vi "test_RK110512Fiber_Spiral.vi"() -> ()   [LabVIEW 2010, in "FPGAWrapperRK110512Fiber_Spiral.lvclass"]
uses:
  FPGAWrapperRK110512Fiber_Spiral.lvclass
  common/arrays/pixel_raw_data_array.ctl
panel:
  out "DAQ loop counter":i32
  out "channel data block":dbl[][](graph)
  out "timed out?":bool
  in  "timeout (ms)":i32
  in  "block size":i32
  in  "number of channels":i32
  out "Pixel dwell time":dbl
  in  "Run":bool
  in  "Cycles per pixel":i32
  in  "Create":bool
  out "FPGAWrapper out":refnum<class "FPGAWrapperRK110512Fiber_Spiral.lvclass">
  in  "Stop":bool
  # "Test VI for FPGAWrapperRK110512Fiber_Spiral"
  # "µs"
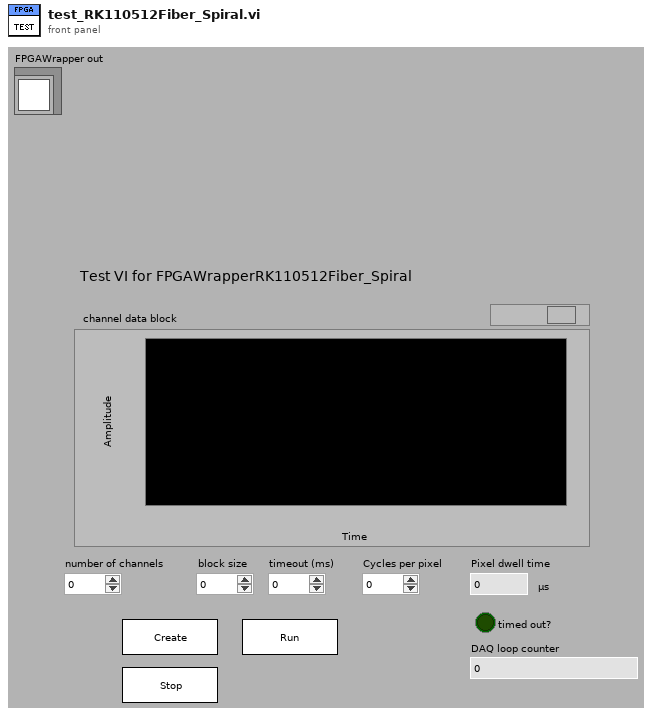
[diagram p1: front panel]
types:
  T1 = typedef "plugin_specification.ctl" = cluster{"class path":string, "configuration":string, "label":string, "settings name":string}
  T2 = typedef "XComponentSpecification.xctl/data.ctl" = cluster{"class path":string, "configuration":string, "label":string, "settings name":string}
  T3 = typedef "pixel_raw_data_array.ctl" = dbl[][]
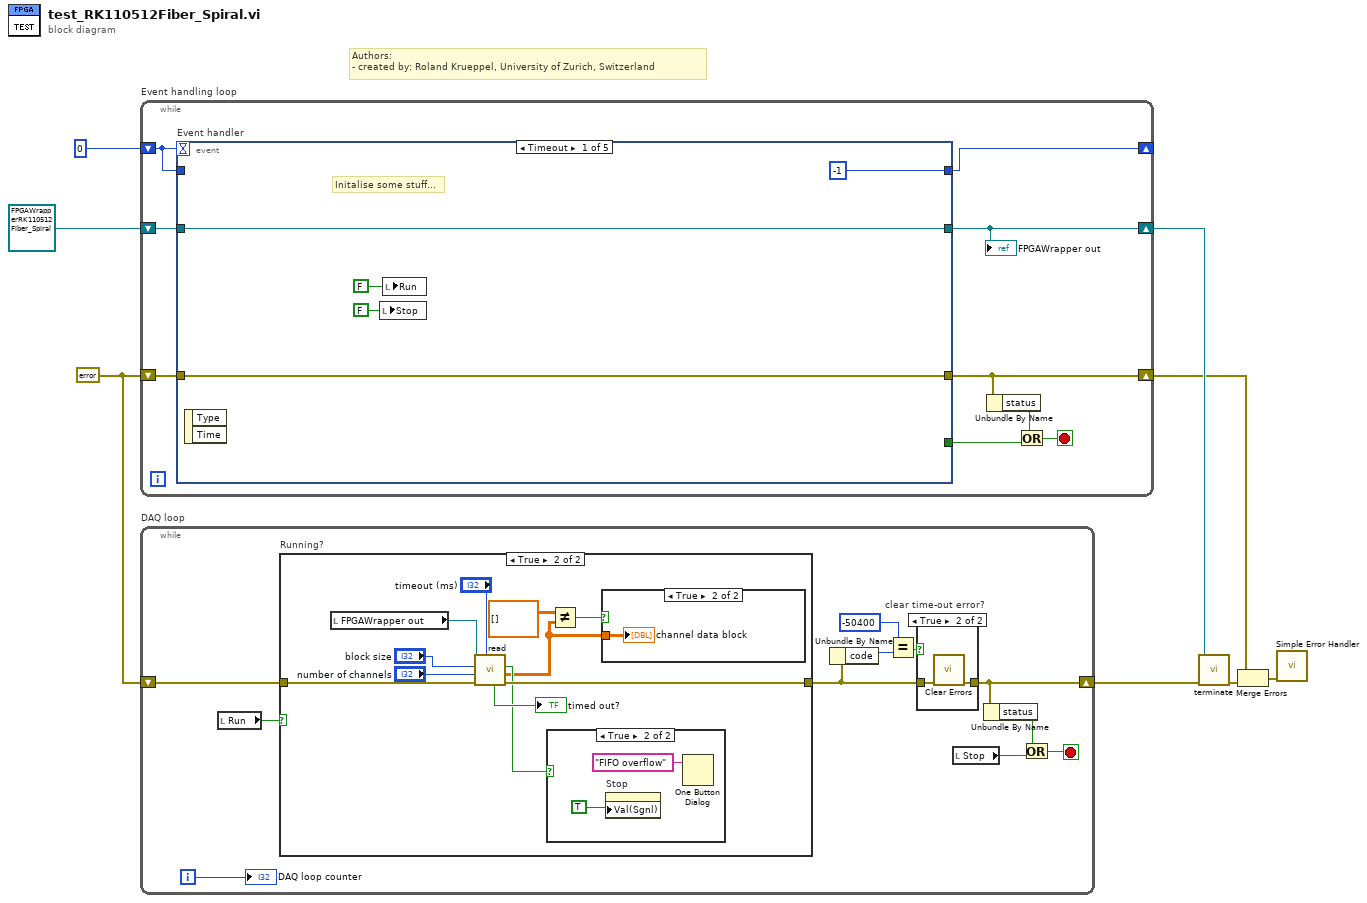
[diagram p0: block diagram]
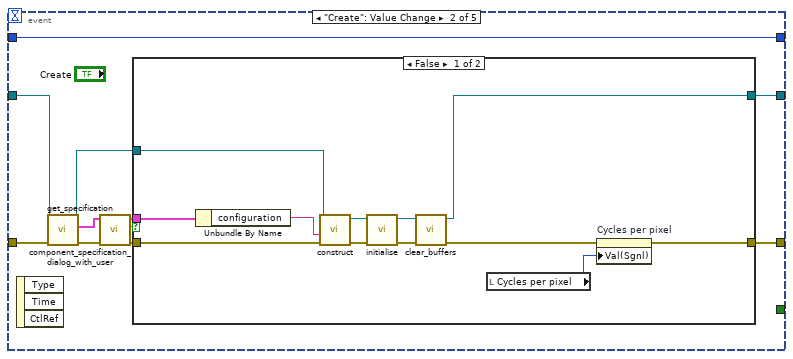
[diagram p6: hidden frame]
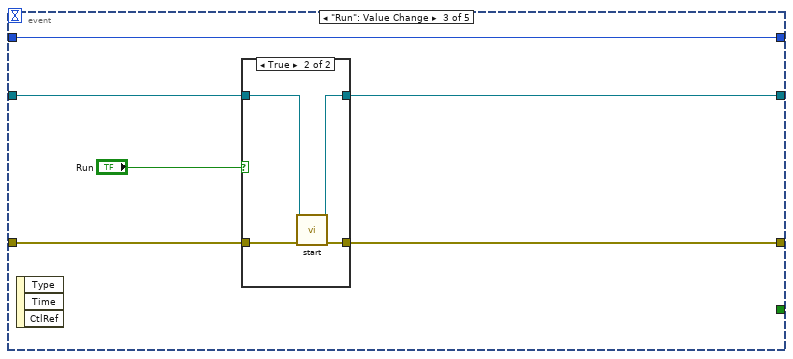
[diagram p8: hidden frame]
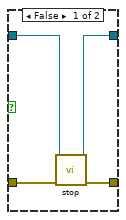
[diagram p9: hidden frame]
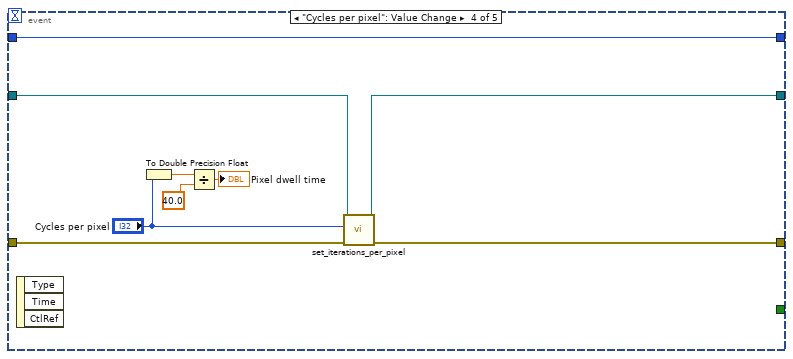
[diagram p10: hidden frame]
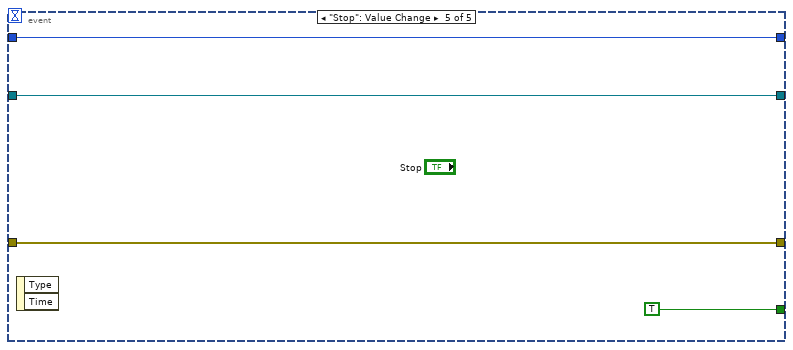
[diagram p11: hidden frame]
diagram:
  w8 = errorcluster {"status"=FALSE, "code"=0, "source"=""} ("error in")
  # "Authors: \n- created by: Roland Krueppel, University of Zurich, Switzerland"
  n1 = while "Event handling loop" {
    shift-right: [w14] -> w2
    shift-left: w8 -> [w17]
    shift-right: [w15] -> _
    shift-left: 0 -> [w16]
    shift-right: [w9] -> w4
    shift-left: refnum<class "FPGAWrapperRK110512Fiber_Spiral.lvclass"> refnum ("FPGAWrapperRK120511Fiber_Spiral.lvclass") -> [w10]
    stop <- w13 stop-if-true
    n2 = event "Event handler" shown="[0] Timeout" {
      selector: _ -> [_ _ _ _ _]
      dyn-events: _ -> [_ _ _ _ _]
      timeout: w16 -> [_ _ _ _ _]
      tunnel: w17 -> [w22 w33 w51 w70 w72]
      tunnel: [w22 w24 w49 w69 w72] -> w14
      tunnel: w16 -> [_ w23 w48 w62 w73]
      tunnel: [-1 w23 w48 w62 w73] -> w15
      tunnel: [_ _ _ _ TRUE ("Stop")] -> w11
      tunnel: w10 -> [w20 w32 w52 w68 w71]
      tunnel: [w20 w25 w50 w67 w71] -> w9
      event Timeout {
        # "Initalise some stuff..."
        n3 = event-data() -> ()  [unwired: 1 in, 2 out]
        n4 = local write "Stop"(FALSE ("Stop")) -> ()
        n5 = local write "Run"(FALSE ("Run")) -> ()
      }
      event "Create": Value Change {
        n6 = event-data() -> ()  [unwired: 1 in, 3 out]
        n7 = call-dynamic "get_specification.vi"("error in (no error)"=w33, "GenericPlugin in"=w32) -> ("error out"=w31:errorcluster, "component specification"=w30:T1, "GenericPlugin out"=w26:refnum<class "FPGAWrapperRK110512Fiber_Spiral.lvclass">)  [unwired: 6 in, 1 out]
        n8 = call "component_specification_dialog_with_user.vi"("error in (no error)"=w31, "component specification in"=w30) -> ("error out"=w28:errorcluster, "cancelled?"=w29:bool, "component specification out"=w27:T2)  [unwired: 7 in]
        n9 = case shown="False" w29 {
          tunnel: w28 -> [w44 w46]
          tunnel: w27 -> [w45 _]
          tunnel: w26 -> [w42 w47]
          tunnel: [w34 w47] -> w25
          tunnel: [w37 w46] -> w24
          frame False {
            n10 = Unbundle By Name(w45) -> ("configuration"=w43:string)
            n11 = call-dynamic "construct.vi"("error in (no error)"=w44, "configuration name"=w43, "GenericPlugin in"=w42) -> ("error out"=w41:errorcluster, "GenericPlugin out"=w40:refnum<class "FPGAWrapperRK110512Fiber_Spiral.lvclass">)  [unwired: 7 in]
            n12 = call-dynamic "initialise.vi"("error in (no error)"=w41, "GenericPlugin in"=w40) -> ("error out"=w39:errorcluster, "GenericPlugin out"=w35:refnum<class "FPGAWrapperRK110512Fiber_Spiral.lvclass">)  [unwired: 8 in]
            n13 = call-dynamic "clear_buffers.vi"("error in (no error)"=w39, "FPGAWrapperRK120511Fiber_Spiral in"=w35) -> ("error out"=w36:errorcluster, "FPGAWrapperRK120511Fiber_Spiral out"=w34:refnum<class "FPGAWrapperRK110512Fiber_Spiral.lvclass">)  [unwired: 8 in]
            n14 = local read "Cycles per pixel"() -> (w38:i32)
            n15 = property on="Cycles per pixel" class="DigNum (strict)"(error in=w36, "Val(Sgnl)"=w38) -> (error out=w37:errorcluster)  [unwired: 1 in, 1 out]
          }
          frame True {
          }
        }
      }
      event "Run": Value Change {
        n16 = event-data() -> ()  [unwired: 1 in, 3 out]
        n17 = case shown="True" "Run" {
          tunnel: w52 -> [w55 w59]
          tunnel: w51 -> [w57 w61]
          tunnel: [w56 w60] -> w49
          tunnel: [w54 w58] -> w50
          frame False {
            n18 = call-dynamic "stop.vi"("error in (no error)"=w57, "FPGAWrapperRK120511Fiber_Spiral in"=w55) -> ("error out"=w56:errorcluster, "FPGAWrapperRK120511Fiber_Spiral out"=w54:refnum<class "FPGAWrapperRK110512Fiber_Spiral.lvclass">)  [unwired: 8 in]
          }
          frame True {
            n19 = call-dynamic "start.vi"("error in (no error)"=w61, "FPGAWrapperRK120511Fiber_Spiral in"=w59) -> ("error out"=w60:errorcluster, "FPGAWrapperRK120511Fiber_Spiral out"=w58:refnum<class "FPGAWrapperRK110512Fiber_Spiral.lvclass">)  [unwired: 8 in]
          }
        }
      }
      event "Cycles per pixel": Value Change {
        n20 = event-data() -> ()  [unwired: 1 in, 3 out]
        n21 = To Double Precision Float(number="Cycles per pixel") -> (double precision float=w65:dbl)
        n22 = Divide(x=w65, y=40.0) -> (x/y=→"Pixel dwell time":dbl)
        n23 = call-dynamic "set_iterations_per_pixel.vi"("error in (no error)"=w70, "iterations per pixel"="Cycles per pixel", "FPGAWrapperRK120511Fiber_Spiral in"=w68) -> ("error out"=w69:errorcluster, "FPGAWrapperRK120511Fiber_Spiral out"=w67:refnum<class "FPGAWrapperRK110512Fiber_Spiral.lvclass">)  [unwired: 7 in]
      }
      event "Stop": Value Change {
        n24 = event-data() -> ()  [unwired: 1 in, 2 out]
      }
    }
    "FPGAWrapper out" <- w9
    n25 = Unbundle By Name(w14) -> ("status"=w12:bool)
    n26 = Or(x=w12, y=w11) -> (x .or. y?=w13:bool)
  }
  n27 = while "DAQ loop" {
    shift-right: [w79] -> w5
    shift-left: w8 -> [w84]
    i -> [w75]
    stop <- w76 stop-if-true
    n28 = local read "Run"() -> (w85:bool)
    n29 = case "Running?" shown="True" w85 {
      tunnel: w84 -> [w89 w100]
      tunnel: [w89 w95] -> w80
      frame False {
      }
      frame True {
        n30 = local read "FPGAWrapper out"() -> (w97:refnum<class "FPGAWrapperRK110512Fiber_Spiral.lvclass">)
        n31 = call-dynamic "read.vi"("timeout (ms)"="timeout (ms)", "error in (no error)"=w100, "number of channels"="number of channels", "block size"="block size", "FPGAWrapperRK120511Fiber_Spiral in"=w97) -> ("error out"=w95:errorcluster, "channels raw data block"=w91:T3, "FIFO full?"=w93:bool, "timed out?"=→"timed out?":bool)  [unwired: 2 in, 1 out]
        n32 = case shown="True" w93 {
          frame False {
          }
          frame True {
            n33 = property on="Stop" class="Bool (strict)"("Val(Sgnl)"=TRUE) -> ()  [unwired: 2 in, 2 out]
            n34 = One Button Dialog(message="FIFO overflow") -> ()  [unwired: 1 in, 1 out]
          }
        }
        n35 = Not Equal?(x=T3 [], y=w91) -> (x != y?=w92:bool)
        n36 = case shown="True" w92 {
          tunnel: w91 -> [_ w101]
          frame False {
          }
          frame True {
            "channel data block" <- w101
          }
        }
      }
    }
    n37 = Unbundle By Name(w80) -> ("code"=w83:i32)
    n38 = Equal?(x=-50400, y=w83) -> (x = y?=w81:bool)
    n39 = case "clear time-out error?" shown="True" w81 {
      tunnel: w80 -> [w86 w88]
      tunnel: [w86 w87] -> w79
      frame False {
      }
      frame True {
        n40 = call <vilib>:"Clear Errors.vi"("error in (no error)"=w88) -> ("error out"=w87:errorcluster)  [unwired: 6 out]
      }
    }
    n41 = local read "Stop"() -> (w77:bool)
    n42 = Unbundle By Name(w79) -> ("status"=w78:bool)
    n43 = Or(x=w78, y=w77) -> (x .or. y?=w76:bool)
    "DAQ loop counter" <- w75
  }
  n44 = call-dynamic "terminate.vi"("error in (no error)"=w5, "GenericPlugin in"=w4) -> ("error out"=w3:errorcluster)  [unwired: 8 in, 1 out]
  n45 = Merge Errors(w2, w3) -> (w1:errorcluster)
  n46 = call <vilib>:"Simple Error Handler.vi"("error in (no error)"=w1) -> ()  [unwired: 4 in, 5 out]
